vi "Measurement Logic.vi"() -> ()   [LabVIEW 2024, in "PMIC_Efficiency.lvlib"]
uses:
  PMIC_Efficiency.lvlib
  Measurement Configuration.ctl
  Measurement Results.ctl
  <vilib>/MeasurementLink/MeasurementLink Measurement Server/Measure Call Context/Measure Call Context.lvclass
  <instrlib>/niDCPower/nidcpower.llb/niDCPower Sense.ctl
  <instrlib>/niDCPower/nidcpower.llb/niDCPower Wait For Event - Event.ctl
  <instrlib>/niDCPower/nidcpower.llb/niDCPower Source Mode.ctl
  <instrlib>/niDCPower/nidcpower.llb/niDCPower Output Function.ctl
  <instrlib>/niDCPower/nidcpower.llb/niDCPower Sequence Attribute Type.ctl
  <instrlib>/niDCPower/nidcpower.llb/niDCPower Create Advanced Sequence Step.vi
  <instrlib>/niDCPower/nidcpower.llb/niDCPower Configure Digital Edge Source Trigger.vi
  <instrlib>/niDCPower/nidcpower.llb/niDCPower Configure Digital Edge Measure Trigger.vi
panel:
  out "measure call context out":refnum<class "Measure Call Context.lvclass">
  in  "measure call context in":refnum<class "Measure Call Context.lvclass">
  out "measurement results":T1
  in  "measurement configuration":T2={"Source device name"="PXIe-4151", "Source current limit (A)"=25.0, "Source power boundary (W)"=300.0, "Source values (V)"=[], "Load device name"="PXIe-4051", "Load voltage limit (V)"=6.0, "Sweep type"=1, "Points or Points/Decade"=10, "Current load level start"=0.1, "Current load level stop"=24.0, "Source delay (s)"=0.005, "DUT setup time (s)"=1.0, "Aperture time (s)"=0.005, "Timeout (s)"=15.0} {"Timeout (s)" format="%.3p"; "DUT setup time (s)" format="%.2p"; "Current load level stop" min=0.0 step=0.1; "Current load level start" min=0.0 step=0.1; "Sweep type" items=["Linear", "Logarithmic"]}
  out "error out":errorcluster
  in  "error in":errorcluster
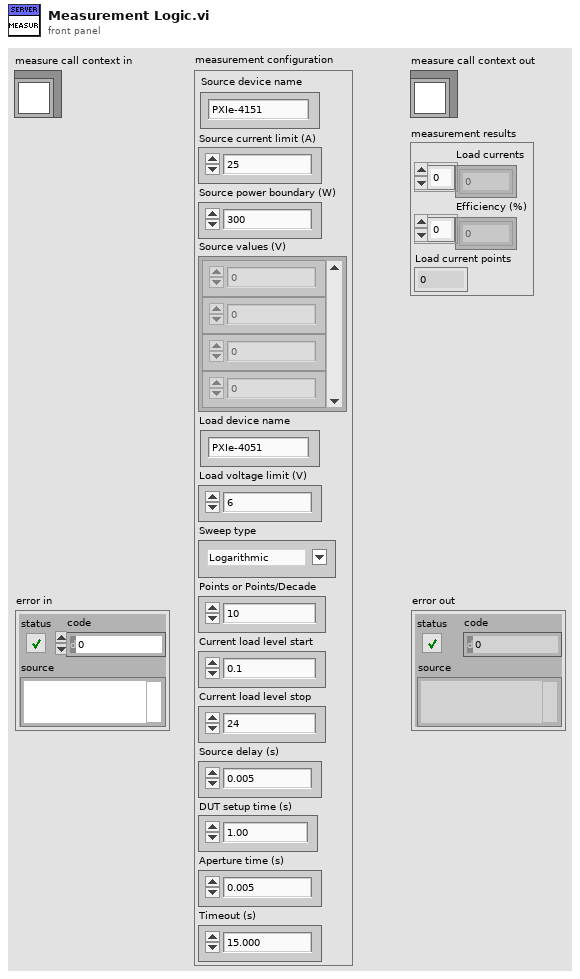
[diagram p1: front panel]
types:
  T1 = typedef "PMIC_Efficiency.lvlib/Measurement Results.ctl" = cluster{"Load currents":dbl[], "Efficiency (%)":dbl[], "Load current points":i32}
  T2 = typedef "PMIC_Efficiency.lvlib/Measurement Configuration.ctl" = cluster{"Source device name":string, "Source current limit (A)":dbl, "Source power boundary (W)":dbl, "Source values (V)":dbl[], "Load device name":string, "Load voltage limit (V)":dbl, "Sweep type":u32, "Points or Points/Decade":i32, "Current load level start":dbl, "Current load level stop":dbl, "Source delay (s)":dbl, "DUT setup time (s)":dbl, "Aperture time (s)":dbl, "Timeout (s)":dbl}
  T3 = cluster{"Source session":refnum<k15>, "Load session":refnum<k15>, "Channel name":string, "Load current points":i32, "Load current levels":dbl[], "Source trigger":string, "Source complete event":string}
  T4 = typedef "niDCPower Source Mode.ctl" = i32
  T5 = typedef "niDCPower Wait For Event - Event.ctl" = i32
  T6 = typedef "niDCPower Sense.ctl" = i32
  T7 = typedef "niDCPower Sequence Attribute Type.ctl" = i32
  T8 = typedef "niDCPower Output Function.ctl" = i32
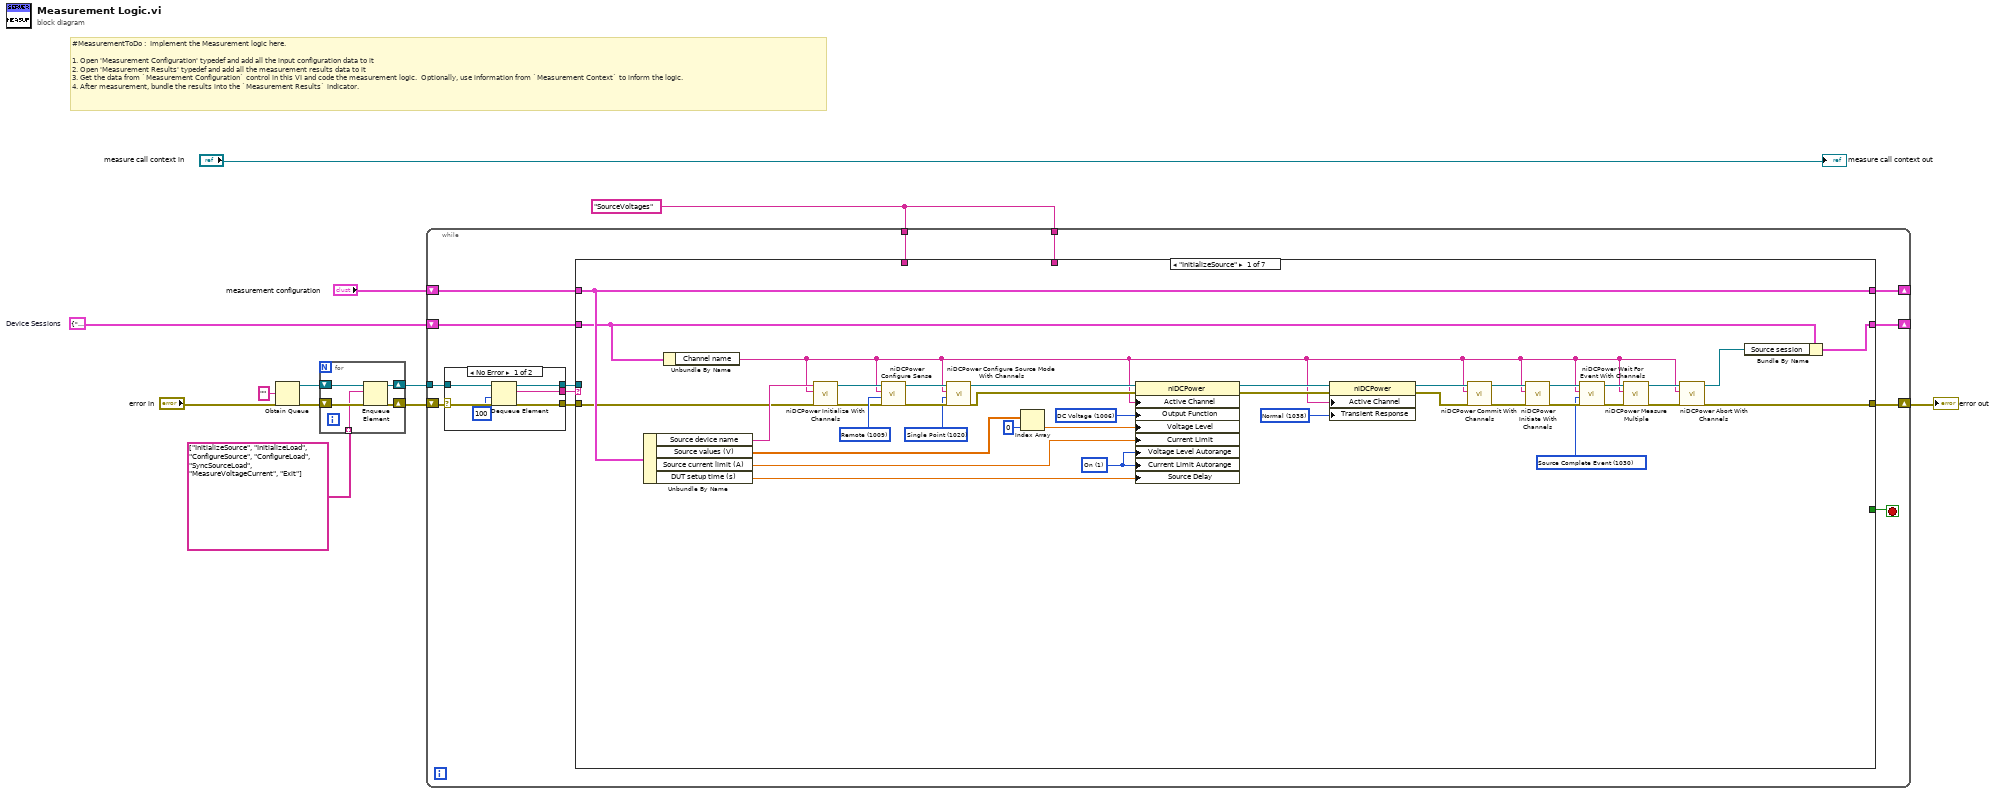
[diagram p0: block diagram]
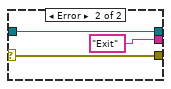
[diagram p2: hidden frame]
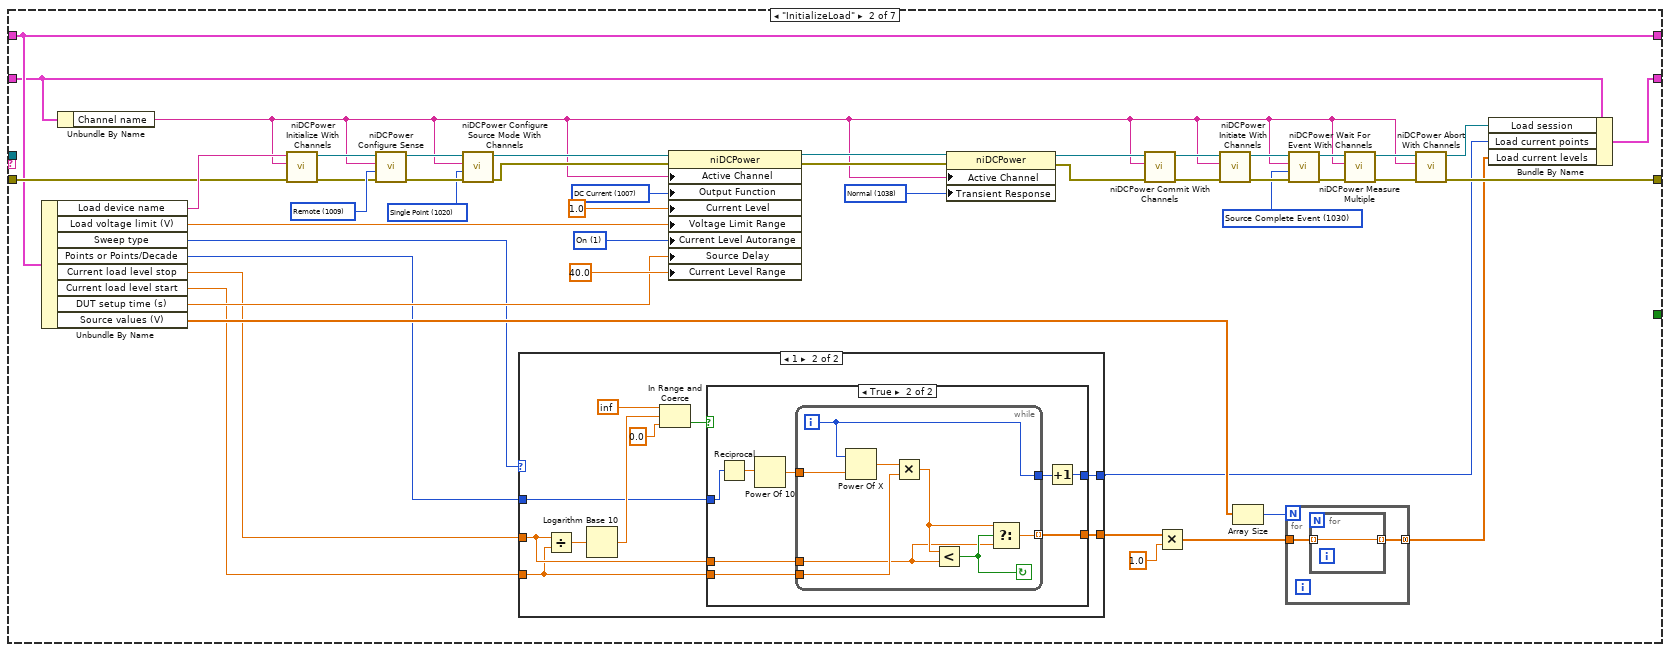
[diagram p3: hidden frame]
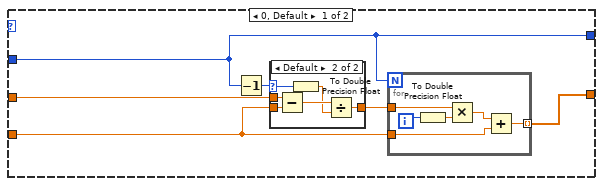
[diagram p4: hidden frame]
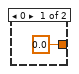
[diagram p5: hidden frame]
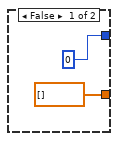
[diagram p6: hidden frame]
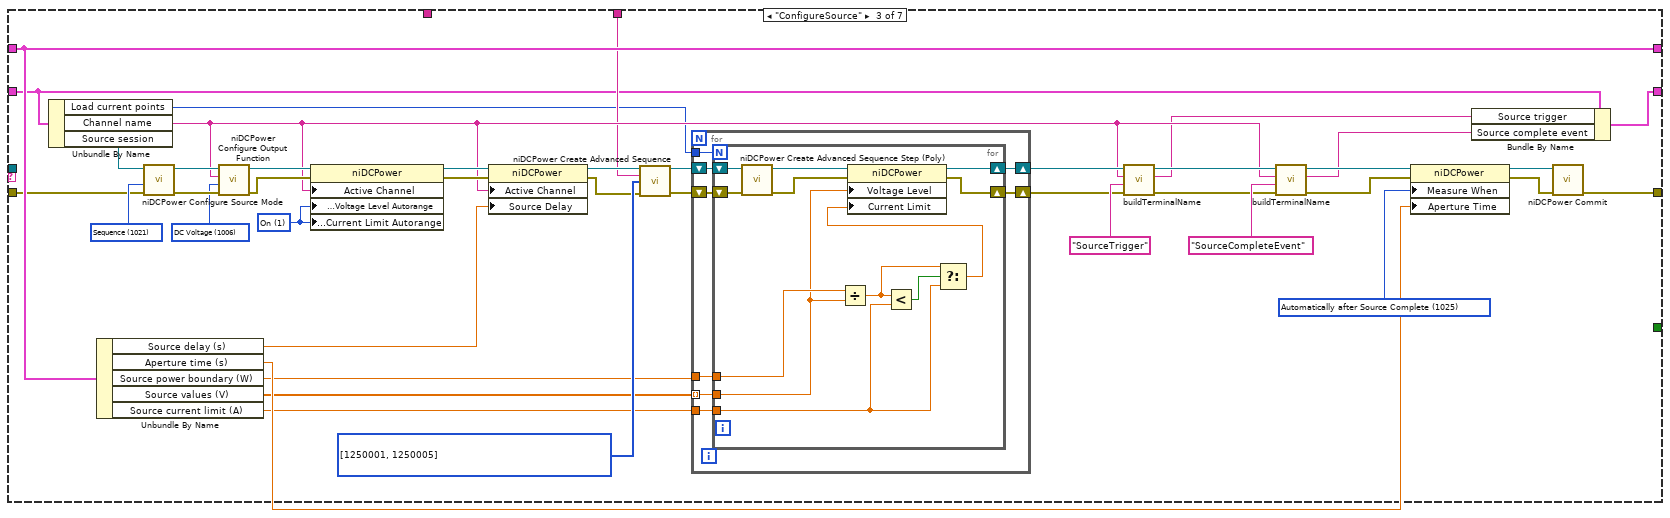
[diagram p7: hidden frame]
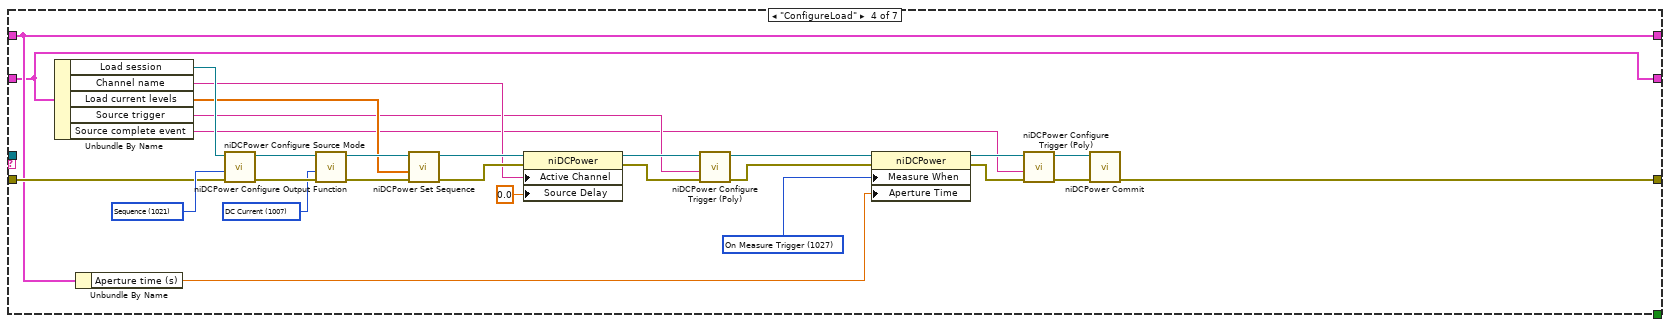
[diagram p8: hidden frame]
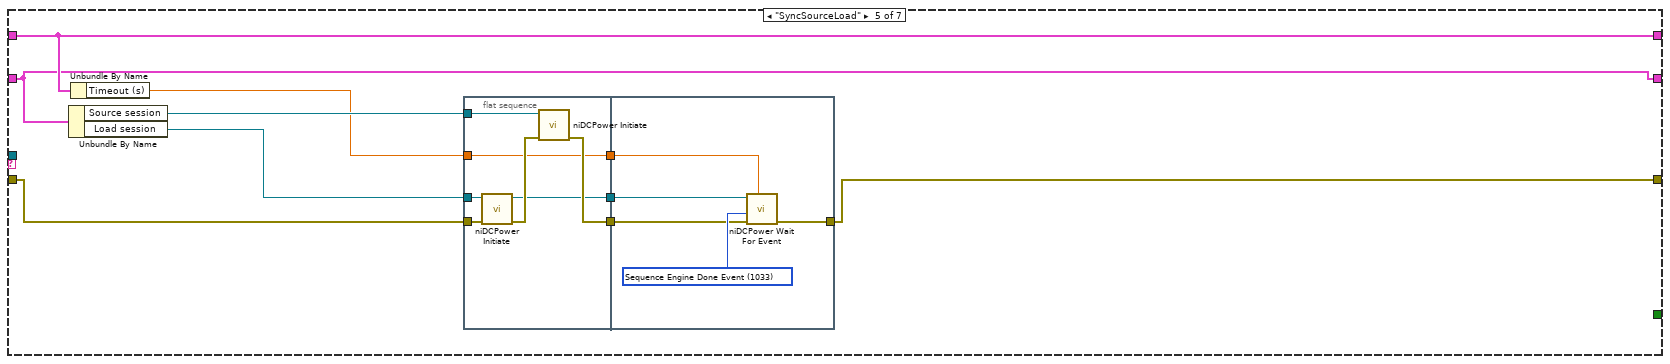
[diagram p9: hidden frame]
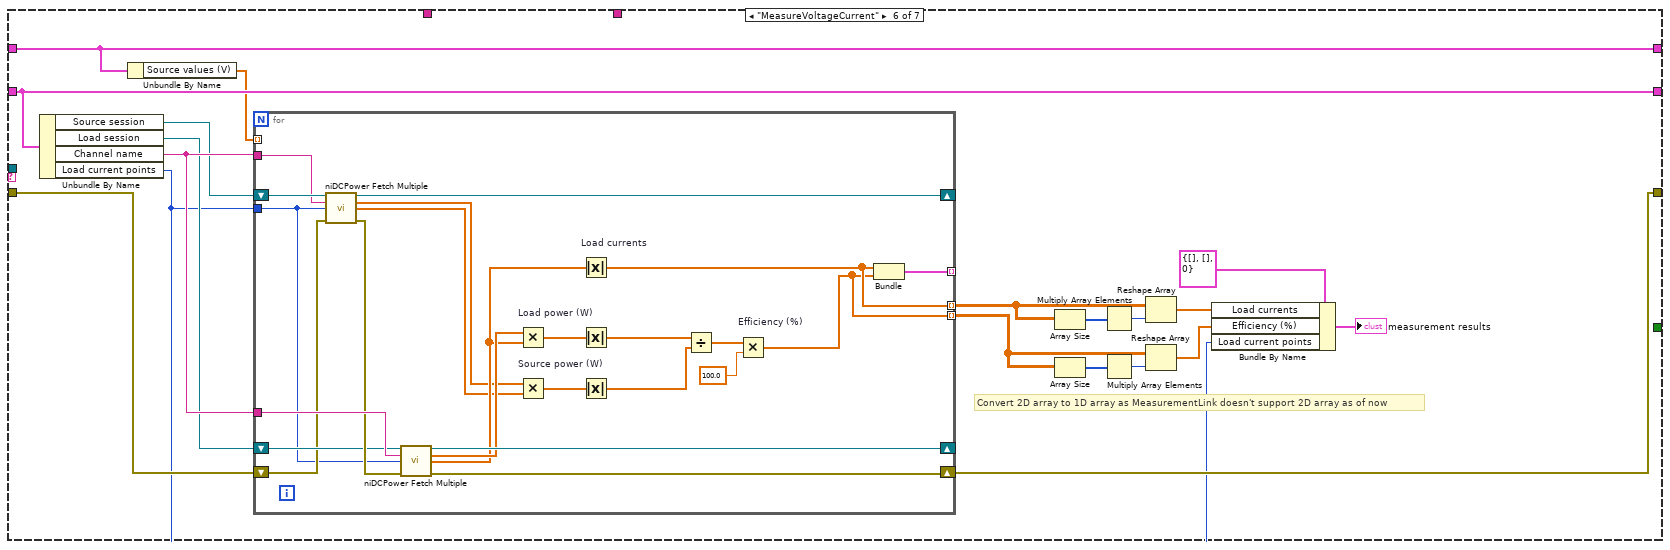
[diagram p10: hidden frame]
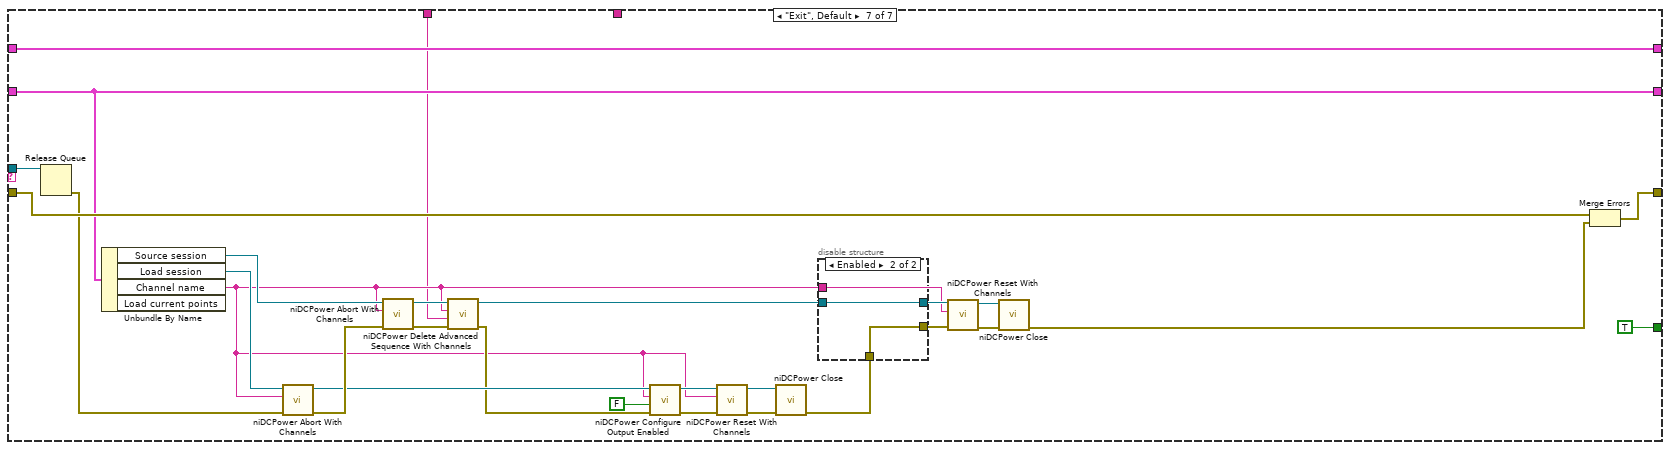
[diagram p11: hidden frame]
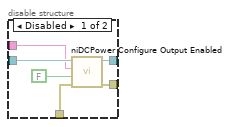
[diagram p12: hidden frame]
diagram:
  w1 = "SourceVoltages" ("sequence name")
  w2 = T3 {"Source session"="", "Load session"="", "Channel name"="0", "Load current points"=0, "Load current levels"=[], "Source trigger"="", "Source complete event"=""}  # Device Sessions
  # "#MeasurementToDo :  Implement the Measurement logic here.\n\n1. Open 'Measurement Configuration' typedef and add all the input configuration data to it\n2. Open 'Measurement Results' typedef and add all the measurement results data to it\n3. Get the data from `Measurement Configuration` control in this VI and code the measurement logic.  Optionally, use information from `Measurement Context` to inform the logic.\n4. After measurement, bundle the results into the `Measurement Results` indicator."
  n1 = Obtain Queue(element data type="", error in (no error)="error in") -> (queue out=w10:refnum<queue>, error out=w7:errorcluster)  [unwired: 3 in, 1 out]
  n2 = for {
    shift-right: [w15] -> w9
    shift-left: w10 -> [w17]
    shift-right: [w14] -> w6
    shift-left: w7 -> [w16]
    tunnel: string[] ["InitializeSource", "InitializeLoad", "ConfigureSource", "ConfigureLoad", "SyncSourceLoad", "MeasureVoltageCurrent", "Exit"] ("Step sequence") -> [w13] mode=indexing
    n3 = Enqueue Element(queue=w17, element=w13, error in (no error)=w16) -> (queue out=w15:refnum<queue>, error out=w14:errorcluster)  [unwired: 1 in, 1 out]
  }
  n4 = while {
    tunnel: w9 -> [w26]
    shift-right: [w30] -> w5
    shift-left: w6 -> [w27]
    shift-right: [w28] -> _
    shift-left: "measurement configuration" -> [w29]
    shift-right: [w22] -> _
    shift-left: w2 -> [w21]
    tunnel: w1 -> [w19]
    tunnel: w1 -> [w18]
    stop <- w23 stop-if-true
    n5 = case shown="No Error" w27 {
      selector: w27 -> [w34 w38]
      tunnel: w26 -> [w36 w37]
      tunnel: [w35 "Exit" ("t")] -> w25
      tunnel: [w31 w38] -> w20
      tunnel: [w32 w37] -> w24
      frame No Error {
        n6 = Dequeue Element(queue=w36, timeout in ms (-1)=100, error in (no error)=w34) -> (queue out=w32:refnum<queue>, element=w35:string, error out=w31:errorcluster)  [unwired: 1 out]
      }
      frame Error {
      }
    }
    n7 = case shown="\"InitializeSource\"" w25 {
      tunnel: [w44 w91 w188 w237 w264 w298 w352] -> w30
      tunnel: w20 -> [w45 w92 w181 w244 w269 w299 w353]
      tunnel: w29 -> [w50 w90 w186 w239 w268 w295 w350]
      tunnel: [w50 w90 w186 w239 w268 w295 w350] -> w28
      tunnel: w24 -> [_ _ _ _ _ _ w354]
      tunnel: [_ _ _ _ _ _ TRUE] -> w23
      tunnel: [w43 w81 w176 w236 w263 w300 w328] -> w22
      tunnel: w21 -> [w40 w80 w177 w236 w263 w300 w328]
      tunnel: w19 -> [_ _ w180 _ _ _ _]
      tunnel: w18 -> [_ _ _ _ _ _ w327]
      frame "InitializeSource" {
        w56 = 1038 items=["Slow"=1041, "Normal"=1038, "Fast"=1039, "Custom"=1042] ("Source:Transient Response")
        w60 = T4 1020 items=["Single Point"=1020, "Sequence"=1021] ("source mode")
        w65 = 1006 items=["DC Voltage"=1006, "DC Current"=1007, "Pulse Voltage"=1049, "Pulse Current"=1050] ("Source:Output Function")
        w70 = T5 1030 items=["Source Complete Event"=1030, "Measure Complete Event"=1031, "Sequence Iteration Complete Event"=1032, "Sequence Engine Done Event"=1033, "Pulse Complete Event"=1051, "Ready For Pulse Trigger Event"=1052] ("event")
        w73 = 1 items=["Off", "On"] ("Source:DC Current:Current Level Autorange")
        w76 = T6 1009 items=["Local"=1008, "Remote"=1009] ("sense")
        n8 = Unbundle By Name(w50) -> ("Source device name"=w51:string, "Source values (V)"=w49:dbl[], "Source current limit (A)"=w47:dbl, "DUT setup time (s)"=w46:dbl)
        n9 = Unbundle By Name(w40) -> ("Channel name"=w41:string)
        n10 = call <instrlib>:"niDCPower Initialize With Channels.vi"("error in (no error)"=w45, "channels"=w41, "resource name"=w51) -> ("error out"=w74:errorcluster, "instrument handle out"=w75:refnum<k15>)  [unwired: 2 in, 5 out]
        n11 = call <instrlib>:"niDCPower Configure Sense.vi"("error in (no error)"=w74, "sense"=w76, "channel name"=w41, "instrument handle"=w75) -> ("error out"=w62:errorcluster, "instrument handle out"=w64:refnum<k15>)  [unwired: 6 in]
        n12 = call <instrlib>:"niDCPower Configure Source Mode With Channels.vi"("error in (no error)"=w62, "source mode"=w60, "channel name"=w41, "instrument handle"=w64) -> ("error out"=w61:errorcluster, "instrument handle out"=w63:refnum<k15>)  [unwired: 6 in]
        n13 = Index Array(array=w49, index=0) -> (element=w48:dbl)
        n14 = property class="niDCPower"(reference=w63, error in=w61, "Active Channel"=w41, "Output Function"=w65, "Voltage Level"=w48, "Current Limit"=w47, "Voltage Level Autorange"=w73, "Current Limit Autorange"=w73, "Source Delay"=w46) -> (reference out=w58:refnum<k15>, error out=w57:errorcluster)
        n15 = property class="niDCPower"(reference=w58, error in=w57, "Active Channel"=w41, "Transient Response"=w56) -> (reference out=w54:refnum<k15>, error out=w55:errorcluster)
        n16 = call <instrlib>:"niDCPower Commit With Channels.vi"("error in (no error)"=w55, "channel name"=w41, "instrument handle"=w54) -> ("error out"=w52:errorcluster, "instrument handle out"=w53:refnum<k15>)  [unwired: 7 in]
        n17 = call <instrlib>:"niDCPower Initiate With Channels.vi"("error in (no error)"=w52, "channel name"=w41, "instrument handle"=w53) -> ("error out"=w72:errorcluster, "instrument handle out"=w71:refnum<k15>)  [unwired: 7 in]
        n18 = call <instrlib>:"niDCPower Wait For Event With Channels.vi"("error in (no error)"=w72, "event"=w70, "channel name"=w41, "instrument handle"=w71) -> ("error out"=w69:errorcluster, "instrument handle out"=w68:refnum<k15>)  [unwired: 6 in]
        n19 = call <instrlib>:"niDCPower Measure Multiple.vi"("error in (no error)"=w69, "channel name"=w41, "instrument handle"=w68) -> ("error out"=w66:errorcluster, "instrument handle out"=w67:refnum<k15>)  [unwired: 5 in, 2 out]
        n20 = call <instrlib>:"niDCPower Abort With Channels.vi"("error in (no error)"=w66, "channel name"=w41, "instrument handle"=w67) -> ("error out"=w44:errorcluster, "instrument handle out"=w42:refnum<k15>)  [unwired: 7 in]
        n21 = Bundle By Name(cluster=w40, "Source session"=w42) -> (w43:T3)
      }
      frame "InitializeLoad" {
        w101 = 1038 items=["Slow"=1041, "Normal"=1038, "Fast"=1039, "Custom"=1042] ("Source:Transient Response")
        w104 = T4 1020 items=["Single Point"=1020, "Sequence"=1021] ("source mode")
        w113 = T5 1030 items=["Source Complete Event"=1030, "Measure Complete Event"=1031, "Sequence Iteration Complete Event"=1032, "Sequence Engine Done Event"=1033, "Pulse Complete Event"=1051, "Ready For Pulse Trigger Event"=1052] ("event")
        w118 = 1 items=["Off", "On"] ("Source:DC Current:Current Level Autorange")
        w119 = 1007 items=["DC Voltage"=1006, "DC Current"=1007, "Pulse Voltage"=1049, "Pulse Current"=1050] ("Source:Output Function")
        w121 = T6 1009 items=["Local"=1008, "Remote"=1009] ("sense")
        n22 = Unbundle By Name(w90) -> ("Load device name"=w95:string, "Load voltage limit (V)"=w87:dbl, "Sweep type"=w86:u32, "Points or Points/Decade"=w85:i32, "Current load level stop"=w84:dbl, "Current load level start"=w83:dbl, "DUT setup time (s)"=w89:dbl, "Source values (V)"=w88:dbl[])
        n23 = Unbundle By Name(w80) -> ("Channel name"=w79:string)
        n24 = call <instrlib>:"niDCPower Initialize With Channels.vi"("error in (no error)"=w92, "channels"=w79, "resource name"=w95) -> ("error out"=w116:errorcluster, "instrument handle out"=w117:refnum<k15>)  [unwired: 2 in, 5 out]
        n25 = call <instrlib>:"niDCPower Configure Sense.vi"("error in (no error)"=w116, "sense"=w121, "channel name"=w79, "instrument handle"=w117) -> ("error out"=w107:errorcluster, "instrument handle out"=w108:refnum<k15>)  [unwired: 6 in]
        n26 = call <instrlib>:"niDCPower Configure Source Mode With Channels.vi"("error in (no error)"=w107, "source mode"=w104, "channel name"=w79, "instrument handle"=w108) -> ("error out"=w105:errorcluster, "instrument handle out"=w106:refnum<k15>)  [unwired: 6 in]
        n27 = case shown="1" w86 {
          tunnel: w85 -> [w127 w146]
          tunnel: [w130 w150] -> w123
          tunnel: w83 -> [w129 w147]
          tunnel: w84 -> [w128 w154]
          tunnel: [w127 w151] -> w78
          frame 0, Default {
            n28 = Decrement(x=w127) -> (x-1=w132:i32)
            n29 = case shown="Default" w132 {
              selector: w132 -> [_ w140]
              tunnel: w128 -> [_ w145]
              tunnel: w129 -> [_ w144]
              tunnel: [0.0 w142] -> w131
              frame 0 {
              }
              frame Default {
                n30 = Subtract(x=w145, y=w144) -> (x-y=w143:dbl)
                n31 = To Double Precision Float(number=w140) -> (double precision float=w141:dbl)
                n32 = Divide(x=w143, y=w141) -> (x/y=w142:dbl)
              }
            }
            n33 = for {
              N: w127 -> [_]
              tunnel: w131 -> [w137]
              tunnel: w129 -> [w138]
              tunnel: [w133] -> w130 mode=indexing
              i -> [w136]
              n34 = To Double Precision Float(number=w136) -> (double precision float=w134:dbl)
              n35 = Multiply(x=w137, y=w134) -> (x*y=w135:dbl)
              n36 = Add(x=w135, y=w138) -> (x+y=w133:dbl)
            }
          }
          frame 1 {
            n37 = Divide(x=w154, y=w147) -> (x/y=w155:dbl)
            n38 = Logarithm Base 10(1:w155) -> (0:w152:dbl)
            n39 = In Range and Coerce(upper limit=inf, x=w152, lower limit=0.0) -> (In Range?=w149:bool)  [unwired: 1 out]
            n40 = case shown="True" w149 {
              tunnel: [dbl[] [] w165] -> w150
              tunnel: [0 w158] -> w151
              tunnel: w154 -> [_ w164]
              tunnel: w147 -> [_ w163]
              tunnel: w146 -> [_ w160]
              frame False {
              }
              frame True {
                n41 = Reciprocal(x=w160) -> (1/x=w162:dbl)
                n42 = Power Of 10(x=w162) -> (10^x=w161:dbl)
                n43 = while {
                  tunnel: w161 -> [w170]
                  tunnel: w163 -> [w173]
                  tunnel: [w169] -> w165 mode=indexing
                  tunnel: [w171] -> w159
                  tunnel: w164 -> [w166]
                  i -> [w171]
                  stop <- w168 continue-if-true
                  n44 = Power Of X(1:w170, 2:w171) -> (0:w172:dbl)
                  n45 = Multiply(x=w172, y=w173) -> (x*y=w167:dbl)
                  n46 = Less?(x=w167, y=w166) -> (x < y?=w168:bool)
                  n47 = Select(t=w167, s=w168, f=w166) -> (s? t:f=w169:dbl)
                }
                n48 = Increment(x=w159) -> (x+1=w158:i32)
              }
            }
          }
        }
        n49 = property class="niDCPower"(reference=w106, error in=w105, "Active Channel"=w79, "Output Function"=w119, "Current Level"=1.0 ("Source:DC Current:Current Level"), "Voltage Limit Range"=w87, "Current Level Autorange"=w118, "Source Delay"=w89, "Current Level Range"=40.0 ("Source:DC Current:Current Level Range")) -> (reference out=w103:refnum<k15>, error out=w102:errorcluster)
        n50 = property class="niDCPower"(reference=w103, error in=w102, "Active Channel"=w79, "Transient Response"=w101) -> (reference out=w98:refnum<k15>, error out=w97:errorcluster)
        n51 = call <instrlib>:"niDCPower Commit With Channels.vi"("error in (no error)"=w97, "channel name"=w79, "instrument handle"=w98) -> ("error out"=w100:errorcluster, "instrument handle out"=w99:refnum<k15>)  [unwired: 7 in]
        n52 = Multiply(x=w123, y=1.0) -> (x*y=w120:dbl[])
        n53 = call <instrlib>:"niDCPower Initiate With Channels.vi"("error in (no error)"=w100, "channel name"=w79, "instrument handle"=w99) -> ("error out"=w115:errorcluster, "instrument handle out"=w114:refnum<k15>)  [unwired: 7 in]
        n54 = Array Size(array=w88) -> (size(s)=w96:i32)
        n55 = for {
          N: w96 -> [_]
          tunnel: w120 -> [w125]
          tunnel: [w124] -> w77 mode=concatenating
          n56 = for {
            tunnel: w125 -> [w126] mode=indexing
            tunnel: [w126] -> w124 mode=indexing
          }
        }
        n57 = call <instrlib>:"niDCPower Wait For Event With Channels.vi"("error in (no error)"=w115, "event"=w113, "channel name"=w79, "instrument handle"=w114) -> ("error out"=w112:errorcluster, "instrument handle out"=w111:refnum<k15>)  [unwired: 6 in]
        n58 = call <instrlib>:"niDCPower Measure Multiple.vi"("error in (no error)"=w112, "channel name"=w79, "instrument handle"=w111) -> ("error out"=w109:errorcluster, "instrument handle out"=w110:refnum<k15>)  [unwired: 5 in, 2 out]
        n59 = call <instrlib>:"niDCPower Abort With Channels.vi"("error in (no error)"=w109, "channel name"=w79, "instrument handle"=w110) -> ("error out"=w91:errorcluster, "instrument handle out"=w82:refnum<k15>)  [unwired: 7 in]
        n60 = Bundle By Name(cluster=w80, "Load session"=w82, "Load current points"=w78, "Load current levels"=w77) -> (w81:T3)
      }
      frame "ConfigureSource" {
        w203 = 1 items=["Off", "On"] ("DC Voltage:Voltage Level Autorange")
        w204 = T7[] [1250001, 1250005] items=["Source -> Output Function"=1150008, "Source -> Output Enabled"=1250006, "Source -> Output Resistance"=1150061, "Source -> Transient Response"=1150062, "Source -> Custom Transient Response -> Voltage Gain Bandwidth"=1150067, "Source -> Custom Transient Response -> Voltage Compensation Frequency"=1150068, "Source -> Custom Transient Response -> Voltage Pole-Zero Ratio"=1150069, "Source -> Custom Transient Response -> Current Gain Bandwidth"=1150070, "Source -> Custom Transient Response -> Current Compensation Frequency"=1150071, "Source -> Custom Transient Response -> Current Pole-Zero Ratio"=1150072, "Source -> DC Voltage -> Voltage Level"=1250001, "Source -> DC Voltage -> Voltage Level Range"=1150005, "Source -> DC Voltage -> Current Limit"=1250005, "Source -> DC Voltage -> Current Limit High"=1150187, "Source -> DC Voltage -> Current Limit Low"=1150188, "Source -> DC Voltage -> Current Limit Range"=1150004, "Source -> DC Current -> Current Level"=1150009, "Source -> DC Current -> Current Level Range"=1150011, "Source -> DC Current -> Voltage Limit"=1150010, "Source -> DC Current -> Voltage Limit High"=1150185, "Source -> DC Current -> Voltage Limit Low"=1150186, "Source -> DC Current -> Voltage Limit Range"=1150012, "Source -> Pulse Voltage -> Pulse Voltage Level"=1150080, "Source -> Pulse Voltage -> Pulse Bias Voltage Level"=1150082, "Source -> Pulse Voltage -> Pulse Voltage Level Range"=1150084, "Source -> Pulse Voltage -> Pulse Current Limit"=1150081, "Source -> Pulse Voltage -> Pulse Current Limit High"=1150193, "Source -> Pulse Voltage -> Pulse Current Limit Low"=1150194, "Source -> Pulse Voltage -> Pulse Bias Current Limit"=1150083, "Source -> Pulse Voltage -> Pulse Bias Current Limit High"=1150195, "Source -> Pulse Voltage -> Pulse Bias Current Limit Low"=1150196, "Source -> Pulse Voltage -> Pulse Current Limit Range"=1150085, "Source -> Pulse Current -> Pulse Current Level"=1150086, "Source -> Pulse Current -> Pulse Bias Current Level"=1150088, "Source -> Pulse Current -> Pulse Current Level Range"=1150090, "Source -> Pulse Current -> Pulse Voltage Limit"=1150087, "Source -> Pulse Current -> Pulse Voltage Limit High"=1150189, "Source -> Pulse Current -> Pulse Voltage Limit Low"=1150190, "Source -> Pulse Current -> Pulse Bias Voltage Limit"=1150089, "Source -> Pulse Current -> Pulse Bias Voltage Limit High"=1150191, "Source -> Pulse Current -> Pulse Bias Voltage Limit Low"=1150192, "Source -> Pulse Current -> Pulse Voltage Limit Range"=1150091, "Source -> Advanced -> Source Delay"=1150051, "Source -> Advanced -> Pulse Bias Delay"=1150092, "Source -> Advanced -> Pulse On Time"=1150093, "Source -> Advanced -> Pulse Off Time"=1150094, "Source -> Advanced -> OVP Enabled"=1250002, "Source -> Advanced -> OVP Limit"=1250003, "Source -> Advanced -> Compliance Limit Symmetry"=1150184, "Source -> Advanced -> Sequence Step Delta Time"=1150198, "Measurement -> Sense"=1150013, "Measurement -> Aperture Time"=1150058, "Measurement -> Measure Record Length"=1150063, "Measurement -> Advanced -> DC Noise Rejection"=1150066, "Measurement -> Autorange"=1150244, "Measurement -> Advanced -> Autorange Behavior"=1150245, "Measurement -> Advanced -> Autorange Aperture Time Mode"=1150246, "Measurement -> Advanced -> Autorange Minimum Aperture Time"=1150247, "Measurement -> Advanced -> Autorange Minimum Aperture Time Units"=1150248, "Measurement -> Advanced -> Autorange Minimum Current Range"=1150255, "Measurement -> Advanced -> Autorange Minimum Voltage Range"=1150256, "Measurement -> Advanced -> Autorange Threshold Mode"=1150257, "Measurement -> Advanced -> Autorange Maximum Delay After Range Change"=1150322, "LCR -> Instrument Mode"=1150208, "LCR -> LCR Stimulus Function"=1150209, "LCR -> LCR Frequency"=1150210, "LCR -> LCR Voltage Amplitude"=1150211, "LCR -> LCR Current Amplitude"=1150212, "LCR -> LCR DC Bias Source"=1150213, "LCR -> LCR DC Bias Voltage Level"=1150214, "LCR -> LCR DC Bias Current Level"=1150215, "LCR -> LCR Impedance Autorange"=1150216, "LCR -> LCR Impedance Range"=1150217, "LCR -> LCR Measurement Time"=1150218, "LCR -> LCR Custom Measurement Time"=1150258, "LCR -> LCR Source Delay Mode"=1150315, "LCR -> Compensation -> Open -> Enabled"=1150220, "LCR -> Compensation -> Open -> Conductance"=1150261, "LCR -> Compensation -> Open -> Susceptance"=1150262, "LCR -> Compensation -> Short -> Enabled"=1150221, "LCR -> Compensation -> Short -> Resistance"=1150263, "LCR -> Compensation -> Short -> Reactance"=1150264, "LCR -> Compensation -> Load -> Enabled"=1150222, "LCR -> Compensation -> Load -> Measured Resistance"=1150268, "LCR -> Compensation -> Load -> Measured Reactance"=1150269, "LCR -> Compensation -> Load -> Actual Resistance"=1150270, "LCR -> Compensation -> Load -> Actual Reactance"=1150271] ("advanced sequence properties")
        w207 = T8 1006 items=["DC Voltage"=1006, "DC Current"=1007, "Pulse Voltage"=1049, "Pulse Current"=1050] ("output function")
        w198 = 1025 items=["Automatically after Source Complete"=1025, "On Demand"=1026, "On Measure Trigger"=1027] ("Measurement:Advanced:Measure When")
        w212 = T4 1021 items=["Single Point"=1020, "Sequence"=1021] ("source mode")
        n61 = Unbundle By Name(w177) -> ("Load current points"=w179:i32, "Channel name"=w187:string, "Source session"=w178:refnum<k15>)
        n62 = Unbundle By Name(w186) -> ("Source delay (s)"=w195:dbl, "Aperture time (s)"=w185:dbl, "Source power boundary (W)"=w184:dbl, "Source values (V)"=w183:dbl[], "Source current limit (A)"=w182:dbl)
        n63 = call <instrlib>:"niDCPower Configure Source Mode.vi"("error in (no error)"=w181, "source mode"=w212, "instrument handle"=w178) -> ("error out"=w214:errorcluster, "instrument handle out"=w213:refnum<k15>)  [unwired: 7 out]
        n64 = call <instrlib>:"niDCPower Configure Output Function.vi"("error in (no error)"=w214, "output function"=w207, "channel name"=w187, "instrument handle"=w213) -> ("error out"=w199:errorcluster, "instrument handle out"=w200:refnum<k15>)  [unwired: 6 out]
        n65 = property class="niDCPower"(reference=w200, error in=w199, "Active Channel"=w187, "Source:DC Voltage:Voltage Level Autorange"=w203, "Source:DC Voltage:Current Limit Autorange"=w203) -> (reference out=w202:refnum<k15>, error out=w201:errorcluster)
        n66 = property class="niDCPower"(reference=w202, error in=w201, "Active Channel"=w187, "Source Delay"=w195) -> (reference out=w190:refnum<k15>, error out=w189:errorcluster)
        n67 = call <instrlib>:"niDCPower Create Advanced Sequence.vi"("instrument handle"=w190, "sequence name"=w180, "advanced sequence properties"=w204, "error in (no error)"=w189) -> ("instrument handle out"=w206:refnum<k15>, "error out"=w205:errorcluster)  [unwired: 10 in]
        n68 = for {
          tunnel: w184 -> [w218]
          tunnel: w182 -> [w217]
          tunnel: w183 -> [w216] mode=indexing
          shift-right: [w220] -> w194
          shift-left: w206 -> [w222]
          shift-right: [w219] -> w193
          shift-left: w205 -> [w221]
          tunnel: w179 -> [w215]
          n69 = for {
            N: w215 -> [_]
            shift-right: [w231] -> w219
            shift-left: w221 -> [w234]
            shift-right: [w230] -> w220
            shift-left: w222 -> [w229]
            tunnel: w218 -> [w228]
            tunnel: w216 -> [w223]
            tunnel: w217 -> [w226]
            n70 = call-poly <instrlib>:"niDCPower Create Advanced Sequence Step (Poly).vi"("error in (no error)"=w234, "instrument handle"=w229) -> ("error out"=w232:errorcluster, "instrument handle out"=w233:refnum<k15>)  [unwired: 8 in]
            n71 = Divide(x=w228, y=w223) -> (x/y=w225:dbl)
            n72 = Less?(x=w225, y=w226) -> (x < y?=w227:bool)
            n73 = Select(t=w225, s=w227, f=w226) -> (s? t:f=w224:dbl)
            n74 = property class="niDCPower"(reference=w233, error in=w232, "Voltage Level"=w223, "Current Limit"=w224) -> (reference out=w230:refnum<k15>, error out=w231:errorcluster)
          }
        }
        n75 = call "buildTerminalName.vi"("error in (no error)"=w193, "Local Terminal Name"="SourceTrigger", "Channel Name"=w187, "session handle"=w194) -> ("error IO"=w191:errorcluster, "Fully Qualified Terminal Name"=w175:string, "session handle 2"=w192:refnum<k15>)  [unwired: 5 in]
        n76 = call "buildTerminalName.vi"("error in (no error)"=w191, "Local Terminal Name"="SourceCompleteEvent", "Channel Name"=w187, "session handle"=w192) -> ("error IO"=w196:errorcluster, "Fully Qualified Terminal Name"=w174:string, "session handle 2"=w197:refnum<k15>)  [unwired: 5 out]
        n77 = property class="niDCPower"(reference=w197, error in=w196, "Measure When"=w198, "Aperture Time"=w185) -> (reference out=w211:refnum<k15>, error out=w210:errorcluster)
        n78 = Bundle By Name(cluster=w177, "Source trigger"=w175, "Source complete event"=w174) -> (w176:T3)
        n79 = call <instrlib>:"niDCPower Commit.vi"("error in (no error)"=w210, "instrument handle"=w211) -> ("error out"=w188:errorcluster)  [unwired: 9 out]
      }
      frame "ConfigureLoad" {
        w254 = T8 1007 items=["DC Voltage"=1006, "DC Current"=1007, "Pulse Voltage"=1049, "Pulse Current"=1050] ("output function")
        w255 = 1027 items=["Automatically after Source Complete"=1025, "On Demand"=1026, "On Measure Trigger"=1027] ("Measurement:Advanced:Measure When")
        w256 = T4 1021 items=["Single Point"=1020, "Sequence"=1021] ("source mode")
        n80 = Unbundle By Name(w236) -> ("Load session"=w243:refnum<k15>, "Channel name"=w242:string, "Load current levels"=w241:dbl[], "Source trigger"=w240:string, "Source complete event"=w235:string)
        n81 = Unbundle By Name(w239) -> ("Aperture time (s)"=w238:dbl)
        n82 = call <instrlib>:"niDCPower Configure Source Mode.vi"("error in (no error)"=w244, "source mode"=w256, "instrument handle"=w243) -> ("error out"=w258:errorcluster, "instrument handle out"=w257:refnum<k15>)  [unwired: 7 out]
        n83 = call <instrlib>:"niDCPower Configure Output Function.vi"("error in (no error)"=w258, "output function"=w254, "instrument handle"=w257) -> ("error out"=w245:errorcluster, "instrument handle out"=w246:refnum<k15>)  [unwired: 1 in, 6 out]
        n84 = call <instrlib>:"niDCPower Set Sequence.vi"("error in (no error)"=w245, "values"=w241, "instrument handle"=w246) -> ("error out"=w250:errorcluster, "instrument handle out"=w251:refnum<k15>)  [unwired: 2 in, 5 out]
        n85 = property class="niDCPower"(reference=w251, error in=w250, "Active Channel"=w242, "Source Delay"=0.0 ("Source:Advanced:Source Delay")) -> (reference out=w253:refnum<k15>, error out=w252:errorcluster)
        n86 = call-poly <instrlib>:"niDCPower Configure Trigger (Poly).vi"("error in (no error)"=w252, "input terminal"=w240, "instrument handle"=w253) -> ("error out"=w261:errorcluster, "instrument handle out"=w262:refnum<k15>)  [unwired: 1 in, 6 out]
        n87 = property class="niDCPower"(reference=w262, error in=w261, "Measure When"=w255, "Aperture Time"=w238) -> (reference out=w259:refnum<k15>, error out=w260:errorcluster)
        n88 = call-poly <instrlib>:"niDCPower Configure Trigger (Poly).vi"("error in (no error)"=w260, "input terminal"=w235, "instrument handle"=w259) -> ("error out"=w249:errorcluster, "instrument handle out"=w248:refnum<k15>)  [unwired: 1 in, 6 out]
        n89 = call <instrlib>:"niDCPower Commit.vi"("error in (no error)"=w249, "instrument handle"=w248) -> ("error out"=w237:errorcluster)  [unwired: 9 out]
      }
      frame "SyncSourceLoad" {
        n90 = Unbundle By Name(w263) -> ("Source session"=w267:refnum<k15>, "Load session"=w266:refnum<k15>)
        n91 = Unbundle By Name(w268) -> ("Timeout (s)"=w265:dbl)
        n92 = flat-sequence {
          tunnel: w266 -> [w279]
          tunnel: w269 -> [w278]
          tunnel: w267 -> [w276]
          tunnel: [w275] -> w272
          tunnel: [w274] -> w271
          tunnel: w265 -> [w273]
          tunnel: [w273] -> w270
          tunnel: w272 -> [w283]
          tunnel: w271 -> [w282]
          tunnel: w270 -> [w281]
          tunnel: [w280] -> w264
          frame #0 {
            n93 = call <instrlib>:"niDCPower Initiate.vi"("error in (no error)"=w278, "instrument handle"=w279) -> ("error out"=w277:errorcluster, "instrument handle out"=w274:refnum<k15>)  [unwired: 8 out]
            n94 = call <instrlib>:"niDCPower Initiate.vi"("error in (no error)"=w277, "instrument handle"=w276) -> ("error out"=w275:errorcluster)  [unwired: 9 out]
          }
          frame #1 {
            w284 = T5 1033 items=["Source Complete Event"=1030, "Measure Complete Event"=1031, "Sequence Iteration Complete Event"=1032, "Sequence Engine Done Event"=1033] ("event")
            n95 = call <instrlib>:"niDCPower Wait For Event.vi"("timeout (10.0)"=w281, "error in (no error)"=w283, "event"=w284, "instrument handle"=w282) -> ("error out"=w280:errorcluster)  [unwired: 7 out]
          }
        }
      }
      frame "MeasureVoltageCurrent" {
        # "Convert 2D array to 1D array as MeasurementLink doesn't support 2D array as of now"
        n96 = Unbundle By Name(w300) -> ("Source session"=w302:refnum<k15>, "Load session"=w301:refnum<k15>, "Channel name"=w303:string, "Load current points"=w285:i32)
        n97 = Unbundle By Name(w295) -> ("Source values (V)"=w294:dbl[])
        n98 = for {
          tunnel: w303 -> [w323]
          tunnel: w303 -> [w322]
          shift-right: [w324] -> _
          shift-left: w301 -> [w316]
          shift-right: [w309] -> w298
          shift-left: w299 -> [w315]
          shift-right: [w325] -> _
          shift-left: w302 -> [w326]
          tunnel: w285 -> [w306]
          tunnel: [w314] -> _ mode=indexing
          tunnel: [w308] -> w291 mode=indexing
          tunnel: [w307] -> w287 mode=indexing
          tunnel: w294 -> [_] mode=indexing
          n99 = call <instrlib>:"niDCPower Fetch Multiple.vi"("instrument handle"=w326, "channel name"=w322, "count (1)"=w306, "error in (no error)"=w315) -> ("instrument handle out"=w325:refnum<k15>, "voltage measurements"=w305:dbl[], "current measurements"=w304:dbl[], "error out"=w321:errorcluster)  [unwired: 1 in, 7 out]
          n100 = call <instrlib>:"niDCPower Fetch Multiple.vi"("instrument handle"=w316, "channel name"=w323, "count (1)"=w306, "error in (no error)"=w321) -> ("instrument handle out"=w324:refnum<k15>, "voltage measurements"=w312:dbl[], "current measurements"=w310:dbl[], "error out"=w309:errorcluster)  [unwired: 1 in, 7 out]
          n101 = Multiply "Load power (W)"(x=w312, y=w310) -> (x*y=w320:dbl[])
          n102 = Multiply "Source power (W)"(x=w305, y=w304) -> (x*y=w319:dbl[])
          n103 = Absolute Value "Load currents"(x=w310) -> (abs(x)=w308:dbl[])
          n104 = Absolute Value(x=w320) -> (abs(x)=w311:dbl[])
          n105 = Absolute Value(x=w319) -> (abs(x)=w313:dbl[])
          n106 = Divide(x=w311, y=w313) -> (x/y=w318:dbl[])
          n107 = Multiply "Efficiency (%)"(x=w318, y=100.0) -> (x*y=w307:dbl[])
          n108 = Bundle(w308, w307) -> (w314:cluster{dbl[], dbl[]})  [unwired: 1 out]
        }
        n109 = Array Size(array=w291) -> (size(s)=w293:i32[])
        n110 = Array Size(array=w287) -> (size(s)=w288:i32[])
        n111 = Multiply Array Elements(1:w293) -> (0:w292:i32)
        n112 = Multiply Array Elements(1:w288) -> (0:w289:i32)
        n113 = Reshape Array(w291, w292) -> (w290:dbl[])
        n114 = Reshape Array(w287, w289) -> (w286:dbl[])
        n115 = Bundle By Name(cluster=T1 {"Load currents"=[], "Efficiency (%)"=[], "Load current points"=0} ("Measurement Results"), "Load currents"=w290, "Efficiency (%)"=w286, "Load current points"=w285) -> (→"measurement results":T1)
      }
      frame "Exit", Default {
        n116 = Release Queue(queue=w354) -> (error out=w330:errorcluster)  [unwired: 2 in, 2 out]
        n117 = Unbundle By Name(w328) -> ("Source session"=w336:refnum<k15>, "Load session"=w335:refnum<k15>, "Channel name"=w331:string)  [unwired: 1 out]
        n118 = call <instrlib>:"niDCPower Abort With Channels.vi"("error in (no error)"=w330, "channel name"=w331, "instrument handle"=w335) -> ("error out"=w347:errorcluster, "instrument handle out"=w333:refnum<k15>)  [unwired: 7 in]
        n119 = call <instrlib>:"niDCPower Abort With Channels.vi"("error in (no error)"=w347, "channel name"=w331, "instrument handle"=w336) -> ("error out"=w349:errorcluster, "instrument handle out"=w348:refnum<k15>)  [unwired: 7 in]
        n120 = call <instrlib>:"niDCPower Delete Advanced Sequence With Channels.vi"("error in (no error)"=w349, "sequence name"=w327, "channel name"=w331, "instrument handle"=w348) -> ("error out"=w332:errorcluster, "instrument handle out"=w334:refnum<k15>)  [unwired: 6 in]
        n121 = call <instrlib>:"niDCPower Configure Output Enabled.vi"("error in (no error)"=w332, "output enabled"=FALSE, "channel name"=w331, "instrument handle"=w333) -> ("error out"=w343:errorcluster, "instrument handle out"=w342:refnum<k15>)  [unwired: 6 in]
        n122 = call <instrlib>:"niDCPower Reset With Channels.vi"("error in (no error)"=w343, "channel name"=w331, "instrument handle"=w342) -> ("error out"=w338:errorcluster, "instrument handle out"=w339:refnum<k15>)  [unwired: 7 in]
        n123 = call <instrlib>:"niDCPower Close.vi"("error in (no error)"=w338, "instrument handle"=w339) -> ("error out"=w346:errorcluster)  [unwired: 9 out]
        n124 = disable-structure shown="Enabled" {
          disable-tunnel: w346 -> [w360 w361]
          disable-tunnel: [w359 w361] -> w345
          disable-tunnel: [w358 w362] -> w344
          disable-tunnel: w334 -> [w356 w362]
          disable-tunnel: w331 -> [w355 _]
          frame Disabled {
            n125 = call <instrlib>:"niDCPower Configure Output Enabled.vi"("error in (no error)"=w360, "output enabled"=FALSE, "channel name"=w355, "instrument handle"=w356) -> ("error out"=w359:errorcluster, "instrument handle out"=w358:refnum<k15>)  [unwired: 6 in]
          }
          frame Enabled {
          }
        }
        n126 = call <instrlib>:"niDCPower Reset With Channels.vi"("error in (no error)"=w345, "channel name"=w331, "instrument handle"=w344) -> ("error out"=w341:errorcluster, "instrument handle out"=w340:refnum<k15>)  [unwired: 7 in]
        n127 = call <instrlib>:"niDCPower Close.vi"("error in (no error)"=w341, "instrument handle"=w340) -> ("error out"=w329:errorcluster)  [unwired: 9 out]
        n128 = Merge Errors(w353, w329) -> (w352:errorcluster)
      }
    }
  }
  "error out" <- w5
  "measure call context out" <- "measure call context in"
